vi "Dequeue Results.vi"(11 "Result Model by Reference in":refnum<class "Result Model.lvclass">) -> (3 "Result Model by Reference out":refnum<class "Result Model.lvclass">)   [LabVIEW 2020, in "Result Model.lvclass"]
uses:
  Result Model/Result Model.lvclass
  Result Model/Result Model.lvclass/Result Model.ctl
  <vilib>/Utility/miscctls.llb/LVMapReplaceAction.ctl
  Core/Result/Type.ctl
  Core/Result/Result.lvlib
  Core/Result/Status.ctl
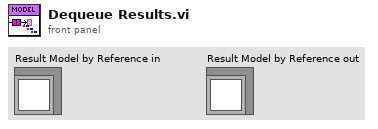
[diagram p1: front panel]
types:
  T1 = typedef "Result.lvlib/Result.ctl" = cluster{"Name":string, "Description":string, "Status":T2, "Result Type":T3, "Execution Time":dbl, "Data":cluster{"Expected":variant, "Actual":variant, "Delta":variant}}
  T2 = typedef "Result.lvlib/Status.ctl" = enum16{"", "Passed", "Failed", "Error", "Skipped", "Setup Error", "Broken", "Teardown Error"}
  T3 = typedef "Result.lvlib/Type.ctl" = enum16{"Test Case", "Test Suite", "Test Run", "Pass", "Fail", "Skip", "Pass if", "Fail if", "Pass if Error", "Fail if Error", "Pass if Equal", "Fail if Equal"}
  T4 = typedef "LVMapReplaceAction.ctl" = enum32{"Modify Entry only if found", "Add or Modify Entry", "Delete Entry"}
  T5 = cluster{"Result Type":T3, "Status":T2, "Description":string, "Data":cluster{"Expected":variant, "Actual":variant, "Delta":variant}}
  T6 = cluster{"Tests":string[], "Run Queue":string[], "Test Statuses":map{string, T2}, "Execution Time":map{string, dbl}, "Assertions":map{string, cluster{"Result Type":T3, "Status":T2, "Description":string, "Data":cluster{"Expected":variant, "Actual":variant, "Delta":variant}}[]}}
  T7 = cluster{"Expected":variant, "Actual":variant, "Delta":variant}
  T8 = map{string, cluster{"Result Type":T3, "Status":T2, "Description":string, "Data":cluster{"Expected":variant, "Actual":variant, "Delta":variant}}[]}
  T9 = cluster{"Result Type":T3, "Status":T2, "Description":string, "Data":cluster{"Expected":variant, "Actual":variant, "Delta":variant}}[]
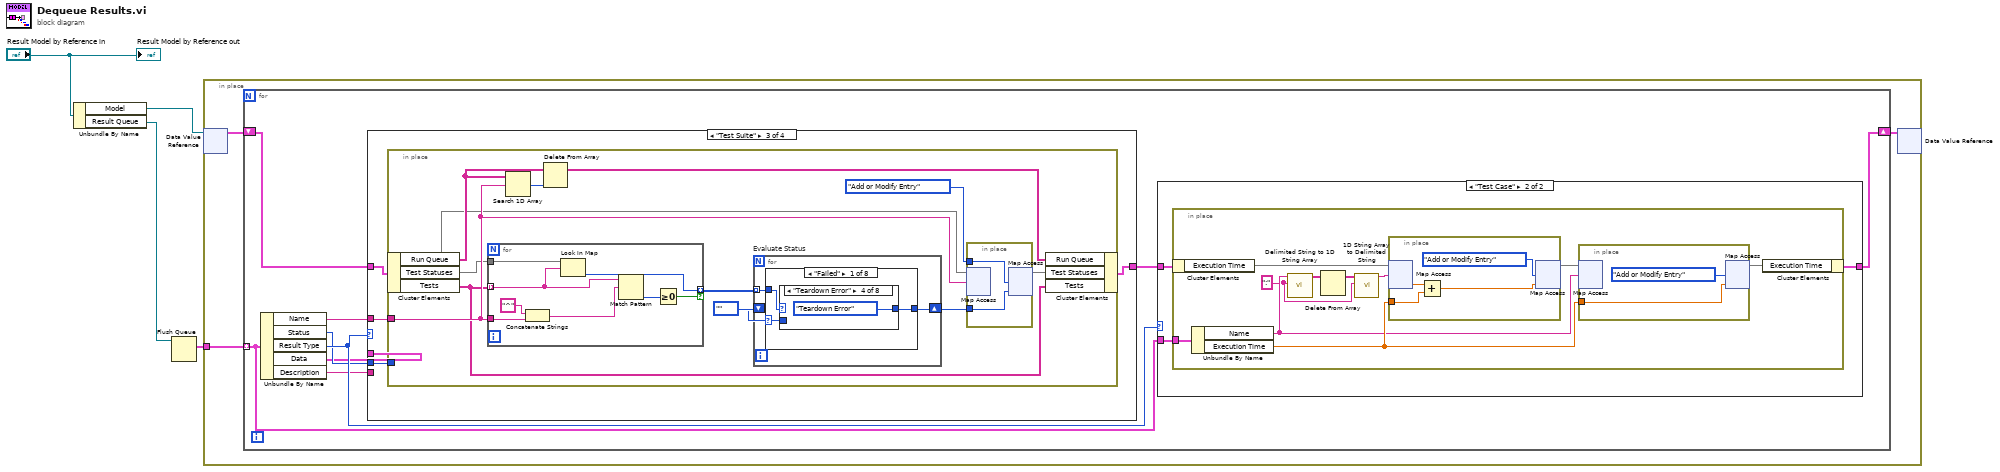
[diagram p0: block diagram]
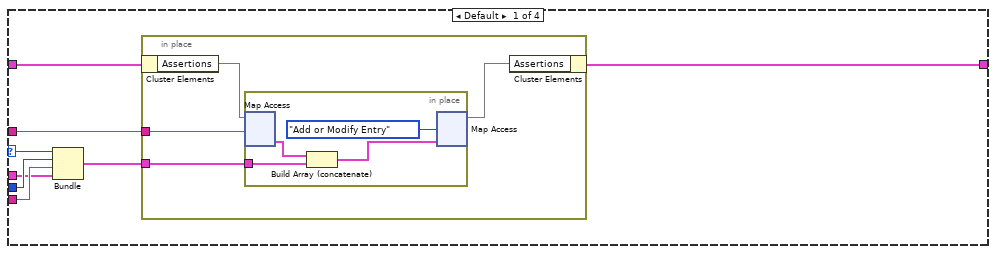
[diagram p2: hidden frame]
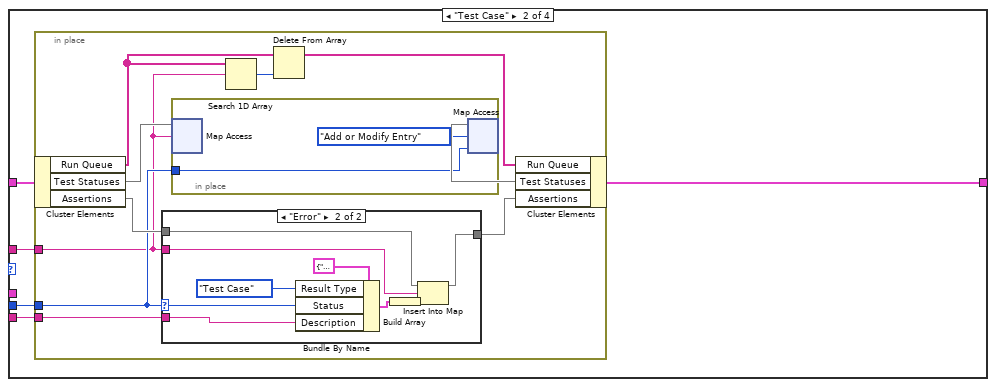
[diagram p3: hidden frame]
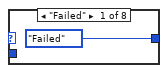
[diagram p5: hidden frame]
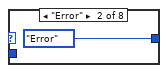
[diagram p6: hidden frame]
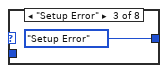
[diagram p7: hidden frame]
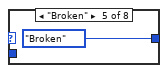
[diagram p8: hidden frame]
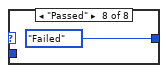
[diagram p11: hidden frame]
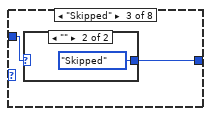
[diagram p13: hidden frame]
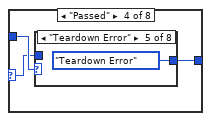
[diagram p15: hidden frame]
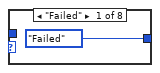
[diagram p16: hidden frame]
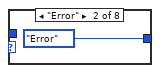
[diagram p17: hidden frame]
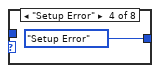
[diagram p19: hidden frame]
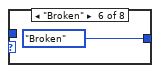
[diagram p20: hidden frame]
diagram:
  n1 = Unbundle By Name("Result Model by Reference in") -> ("Model"=w4:refnum<data-value>, "Result Queue"=w2:refnum<queue>)
  n2 = Flush Queue(queue=w2) -> (remaining elements=w1:T1[])  [unwired: 1 in, 2 out]
  n3 = in-place {
    in-place-border: w1 -> [w5]
    n4 = in-place-dvr #1(w4) -> (w6:T6)  [unwired: 1 out]
    n5 = for {
      shift-right: [w16] -> w7
      shift-left: w6 -> [w15]
      tunnel: w5 -> [w14] mode=indexing
      n6 = Unbundle By Name(w14) -> ("Name"=w12:string, "Status"=w11:T2, "Result Type"=w13:T3, "Data"=w9:T7, "Description"=w10:string)
      n7 = case shown="\"Test Suite\"" w13 {
        selector: w13 -> [w21 _ _ _]
        tunnel: w12 -> [w22 w37 w63 _]
        tunnel: w11 -> [w20 w36 w62 _]
        tunnel: w10 -> [w23 w33 _ _]
        tunnel: w15 -> [w19 w35 w61 w133]
        tunnel: [w18 w34 w60 w133] -> w8
        tunnel: w9 -> [w17 _ _ _]
        frame Default {
          n8 = Bundle("Result Type"=w21, "Status"=w20, "Description"=w23, "Data"=w17) -> (w24:T5)  [unwired: 1 in]
          n9 = in-place {
            in-place-border: w24 -> [w28]
            in-place-border: w22 -> [w27]
            n10 = in-place-cluster #2(w19) -> ("Assertions"=w26:T8)
            n11 = in-place {
              in-place-border: w28 -> [w29]
              n12 = in-place-map #3(w26, w27) -> (w32:T9)  [unwired: 1 in, 1 out]
              n13 = Build Array (concatenate)(w32, w29) -> (w31:T9)
              n14 = in-place-map #3(w31, LVMapReplaceAction."Add or Modify Entry" ("action")) -> (w25:T8)  [unwired: 2 out]
            }
            n15 = in-place-cluster #2("Assertions"=w25) -> (w18:T6)
          }
        }
        frame "Test Case" {
          n16 = in-place {
            in-place-border: w37 -> [w40]
            in-place-border: w36 -> [w43]
            in-place-border: w33 -> [w42]
            n17 = in-place-cluster #4(w35) -> ("Run Queue"=w39:string[], "Test Statuses"=w47:map{string, T2}, "Assertions"=w45:T8)
            n18 = case shown="\"Error\"" w43 {
              selector: w43 -> [_ w53]
              tunnel: w45 -> [w48 w57]
              tunnel: [w48 w56] -> w44
              tunnel: w40 -> [_ w55]
              tunnel: w42 -> [_ w52]
              frame "", Default {
              }
              frame "Error" {
                n19 = Bundle By Name(cluster=T5 {"Result Type"=enum."Test Case", "Status"=enum."", "Description"="", "Data"={"Expected"=variant, "Actual"=variant, "Delta"=variant}} ("value"), "Result Type"=Type."Test Case", "Status"=w53, "Description"=w52) -> (w50:T5)
                n20 = Build Array(w50) -> (w49:T9)
                n21 = Insert Into Map(map in=w57, key=w55, value=w49) -> (map out=w56:T8)  [unwired: 2 out]
              }
            }
            n22 = in-place {
              in-place-border: w43 -> [w58]
              n23 = in-place-map #5(w47, w40) -> ()  [unwired: 1 in, 2 out]
              n24 = in-place-map #5(w58, LVMapReplaceAction."Add or Modify Entry" ("action")) -> (w46:map{string, T2})  [unwired: 2 out]
            }
            n25 = Search 1D Array(1D array=w39, element=w40) -> (index of element=w41:i32)  [unwired: 1 in]
            n26 = Delete From Array(array=w39, index=w41) -> (array with subset deleted=w38:string[])  [unwired: 1 in, 1 out]
            n27 = in-place-cluster #4("Run Queue"=w38, "Test Statuses"=w46, "Assertions"=w44) -> (w34:T6)
          }
        }
        frame "Test Suite" {
          n28 = in-place {
            in-place-border: w63 -> [w66]
            in-place-border: w62 -> [_]
            n29 = in-place-cluster #6(w61) -> ("Run Queue"=w69:string[], "Test Statuses"=w64:map{string, T2}, "Tests"=w65:string[])
            n30 = for {
              tunnel: w66 -> [w82]
              tunnel: [w76] -> w72 mode=indexing if=w80
              tunnel: w65 -> [w75] mode=indexing
              tunnel: w64 -> [w77]
              n31 = Concatenate Strings("^" ("string"), w82) -> (w79:string)
              n32 = Look In Map(map=w77, key=w75) -> (value=w76:T2)  [unwired: 1 in, 1 out]
              n33 = Match Pattern(string=w75, regular expression=w79) -> (offset past match=w81:i32)  [unwired: 1 in, 3 out]
              n34 = Greater Or Equal To 0?(x=w81) -> (x >= 0?=w80:bool)
            }
            n35 = Search 1D Array(1D array=w69, element=w66) -> (index of element=w68:i32)  [unwired: 1 in]
            n36 = Delete From Array(array=w69, index=w68) -> (array with subset deleted=w67:string[])  [unwired: 1 in, 1 out]
            n37 = for "Evaluate Status" {
              tunnel: w72 -> [w83] mode=indexing
              shift-right: [w84] -> w71
              shift-left: Status."" ("Current") -> [w85]
              n38 = case shown="\"Failed\"" w85 {
                selector: w85 -> [w86 _ _ w102 w113 _ _ _]
                tunnel: w83 -> [w88 w97 w98 w104 w114 w119 w123 w127]
                tunnel: [w87 w97 w99 w103 w115 w120 w124 w128] -> w84
                frame "Failed" {
                  n39 = case shown="\"Teardown Error\"" w88 {
                    tunnel: [Status."Failed" ("Merged Status") Status."Error" ("Merged Status") Status."Setup Error" ("Merged Status") Status."Teardown Error" ("Merged Status") Status."Broken" ("Merged Status") w94 w95 Status."Failed" ("Merged Status")] -> w87
                    tunnel: w86 -> [_ _ _ _ _ w94 w95 _]
                    frame "Failed" {
                    }
                    frame "Error" {
                    }
                    frame "Setup Error" {
                    }
                    frame "Teardown Error" {
                    }
                    frame "Broken" {
                    }
                    frame "" {
                    }
                    frame "Skipped" {
                    }
                    frame "Passed" {
                    }
                  }
                }
                frame "" {
                }
                frame "Skipped" {
                  n40 = case shown="\"\"" w98 {
                    selector: w98 -> [w100 _]
                    tunnel: [w100 Status."Skipped" ("Merged Status")] -> w99
                    frame Default {
                    }
                    frame "" {
                    }
                  }
                }
                frame "Passed" {
                  n41 = case shown="\"Teardown Error\"" w104 {
                    tunnel: [Status."Failed" ("Merged Status") Status."Error" ("Merged Status") w107 Status."Setup Error" ("Merged Status") Status."Teardown Error" ("Merged Status") Status."Broken" ("Merged Status") Status."Skipped" ("Merged Status") Status."Passed" ("Merged Status")] -> w103
                    tunnel: w102 -> [_ _ w107 _ _ _ _ _]
                    frame "Failed" {
                    }
                    frame "Error" {
                    }
                    frame "" {
                    }
                    frame "Setup Error" {
                    }
                    frame "Teardown Error" {
                    }
                    frame "Broken" {
                    }
                    frame "Skipped" {
                    }
                    frame "Passed" {
                    }
                  }
                }
                frame "Error" {
                  n42 = case shown="\"Skipped\"" w114 {
                    tunnel: [Status."Skipped" ("Merged Status") w117 Status."Error" ("Merged Status")] -> w115
                    tunnel: w113 -> [_ w117 _]
                    frame "Skipped" {
                    }
                    frame "" {
                    }
                    frame Default {
                    }
                  }
                }
                frame "Setup Error" {
                  n43 = case shown="Default" w119 {
                    tunnel: [Status."Skipped" ("Merged Status") Status."Setup Error" ("Merged Status")] -> w120
                    frame "Skipped" {
                    }
                    frame Default {
                    }
                  }
                }
                frame "Broken" {
                  n44 = case shown="\"Setup Error\"" w123 {
                    tunnel: [Status."Broken" ("Merged Status") Status."Setup Error" ("Merged Status")] -> w124
                    frame Default {
                    }
                    frame "Setup Error" {
                    }
                  }
                }
                frame "Teardown Error" {
                  n45 = case shown="\"Skipped\"" w127 {
                    tunnel: [Status."Skipped" ("Merged Status") Status."Teardown Error" ("Merged Status")] -> w128
                    frame "Skipped" {
                    }
                    frame Default {
                    }
                  }
                }
              }
            }
            n46 = in-place {
              in-place-border: LVMapReplaceAction."Add or Modify Entry" ("action") -> [w132]
              in-place-border: w71 -> [w131]
              n47 = in-place-map #7(w64, w66) -> ()  [unwired: 1 in, 2 out]
              n48 = in-place-map #7(w131, w132) -> (w74:map{string, T2})  [unwired: 2 out]
            }
            n49 = in-place-cluster #6("Run Queue"=w67, "Test Statuses"=w74, "Tests"=w65) -> (w60:T6)
          }
        }
        frame "Test Run" {
        }
      }
      n50 = case shown="\"Test Case\"" w13 {
        tunnel: w14 -> [_ w137]
        tunnel: w8 -> [w134 w135]
        tunnel: [w134 w136] -> w16
        frame Default {
        }
        frame "Test Case" {
          n51 = in-place {
            in-place-border: w137 -> [w146]
            w138 = ":" ("delimiter")
            n52 = in-place-cluster #8(w135) -> ("Execution Time"=w142:map{string, dbl})
            n53 = Unbundle By Name(w146) -> ("Name"=w144:string, "Execution Time"=w145:dbl)
            n54 = call <vilib>:"Delimited String to 1D String Array.vi"("delimiter"=w138, "delimited string"=w144) -> ("string array"=w140:string[])  [unwired: 9 in]
            n55 = Delete From Array(array=w140) -> (array with subset deleted=w139:string[])  [unwired: 2 in, 1 out]
            n56 = call <vilib>:"1D String Array to Delimited String.vi"("delimiter"=w138, "string array"=w139) -> ("delimited string"=w143:string)  [unwired: 9 in]
            n57 = in-place {
              in-place-border: w145 -> [w151]
              n58 = in-place-map #9(w142, w143) -> (w150:dbl)  [unwired: 1 in, 1 out]
              n59 = Add(x=w150, y=w151) -> (x+y=w153:dbl)
              n60 = in-place-map #9(w153, LVMapReplaceAction."Add or Modify Entry" ("action")) -> (w147:map{string, dbl})  [unwired: 2 out]
            }
            n61 = in-place {
              in-place-border: w145 -> [w148]
              n62 = in-place-map #10(w147, w144) -> ()  [unwired: 1 in, 2 out]
              n63 = in-place-map #10(w148, LVMapReplaceAction."Add or Modify Entry" ("action")) -> (w141:map{string, dbl})  [unwired: 2 out]
            }
            n64 = in-place-cluster #8("Execution Time"=w141) -> (w136:T6)
          }
        }
      }
    }
    n65 = in-place-dvr #1(w7) -> ()  [unwired: 2 out]
  }
  "Result Model by Reference out" <- "Result Model by Reference in"
